vi "AOL Control-4ch.vi"() -> ()   [LabVIEW 2020]
uses:
  TypeDef/Frequency-4ch.ctl
  TypeDef/Amplitude-4ch.ctl
  TypeDef/FPGA_card_type.ctl
  TypeDef/FPGA_adapter_type.ctl
  Globals/FPGA Globals.vi
  <vilib>/DAQmx/create/channels.llb/DAQmx Create Channel (CO-Pulse Generation-Time).vi
panel:
  in  "Tab Control":T1(tab)
  out "Continuous Trigger  ON":bool
  in  "Tadj [us]":dbl
  in  "Tdwell [us]":dbl=0.4
  in  "AOD Fill":dbl=24.475
  in  "Ny":u16=39
  in  "Nx":u16=39
  in  "Use Cont. trigger":bool
  in  "Use RF from file":bool
  in  "RF Code File":path=path "D:/Microscope data/2019-04-16/Sameer/Packets"
  in  "Frequency (MHz)":T2={"Ch 1"=39, "Ch 2"=39, "Ch 3"=39, "Ch 4"=39} {"Ch 4" min=20 max=50 step=1; "Ch 3" min=20 max=50 step=1; "Ch 2" min=20 max=50 step=1; "Ch 1" min=20 max=50 step=1}
  in  "Amplitude":T3={"Ch 1"=255, "Ch 2"=255, "Ch 3"=255, "Ch 4"=255} {"Ch 4" max=255 step=1; "Ch 3" max=255 step=1; "Ch 2" max=255 step=1; "Ch 1" max=255 step=1}
  in  "Stop":bool
  in  "Load":bool
  in  "Run":bool
  in  "Clear":bool
  in  "Settings":bool
  out "Ethernet Port Opened":bool
  out "RF Loaded":bool
  out "Trigger Sent":bool
  out "Status":string
  in  "Use detected RIO resource":bool
  in  "RIO Resource Name":string
  out "Detected RIO Resource Name":string
  in  "Use FlexRIO Trigger":bool=TRUE
  in  "DAQmx Trigger Channel":tag="PXI1Slot4/ctr0"
  in  "Pulse Width (sec)":dbl=1e-05
  in  "Initial Delay(sec)":dbl=0.01 format="%.6f"
  in  "FPGA Card":T4
  in  "Adapter Module":T5
  out "task out":refnum<k21>
  out "PC Mac Address":string caption="PC MAC Address"
  out "Select Device 1":i32=1 caption="Device 1 Port" min=1 max=5 step=1
  out "Select Device 2":i32=1 caption="Device 2 Port" min=1 max=5 step=1
  out "Packet Array":string[](array[string])
  out "No of Packets":i32
  out "FPGA MAC 1":string caption="Device 1 MAC Address"
  out "FPGA MAC 2":string caption="Device 2 MAC Address"
  out "Trigger Error":errorcluster
  in  "error in":errorcluster
  # "User needs to send a single TTL rising edge for the controller to generate RF."
  # "Trigger"
  # "Ethernet"
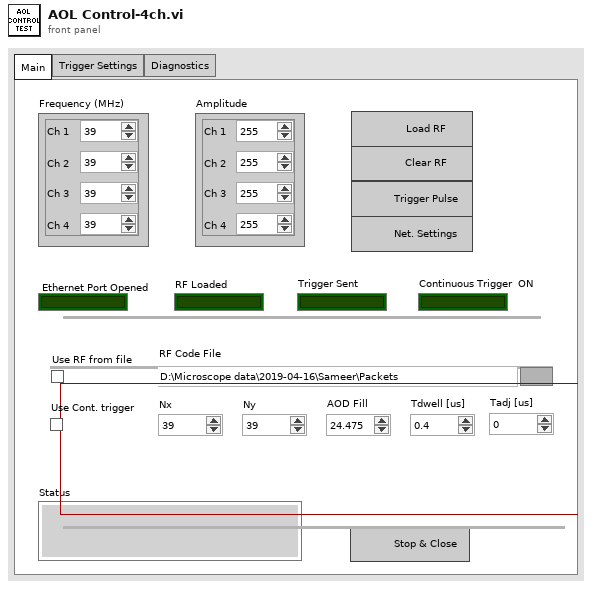
[diagram p1: front panel]
types:
  T1 = enum32{"Main", "Trigger Settings", "Diagnostics"}
  T2 = typedef "Frequency-4ch.ctl" = cluster{"Ch 1":u16, "Ch 2":u16, "Ch 3":u16, "Ch 4":u16}
  T3 = typedef "Amplitude-4ch.ctl" = cluster{"Ch 1":u16, "Ch 2":u16, "Ch 3":u16, "Ch 4":u16}
  T4 = typedef "FPGA_card_type.ctl" = enum16{"7976R", "7975R", "7966R"}
  T5 = typedef "FPGA_adapter_type.ctl" = enum16{"5772-DC", "5772-AC"}
  T6 = enum8{"Enabled", "Disabled", "Disabled and Grayed Out"}
  T7 = enum16{"Initialise FPGA ref", "Read FPGA ref", "Close FPGA Ref"}
  T8 = cluster{"Use FlexRIO Trigger":bool, "RIO Resource Name":string, "Use detected RIO resource":bool, "Ethernet Card WinPCap Port ":i16, "FPGA Card":string, "Adapter Module":string}
  T9 = typedef "FPGA_DAQ_settings.ctl" = cluster{"Use FlexRIO Trigger":bool, "RIO Resource Name":string, "Use detected RIO resource":bool, "Ethernet Card WinPCap Port ":i16, "Adapter Module":T5, "FPGA Card":T4}
  T10 = typedef "FPGA Settings.ctl" = cluster{"System Clock(MHz)":dbl, "FPGA MAC 1":string, "Port Number 1":i32, "Port Number 2":i32, "FPGA MAC 2":string, "PC MAC Address":string}
  T11 = cluster{"Pulse Period (us)":u32, "Pulse Width (us)":u32}
  T12 = typedef "FPGA_ref.ctl" = refnum<k20>
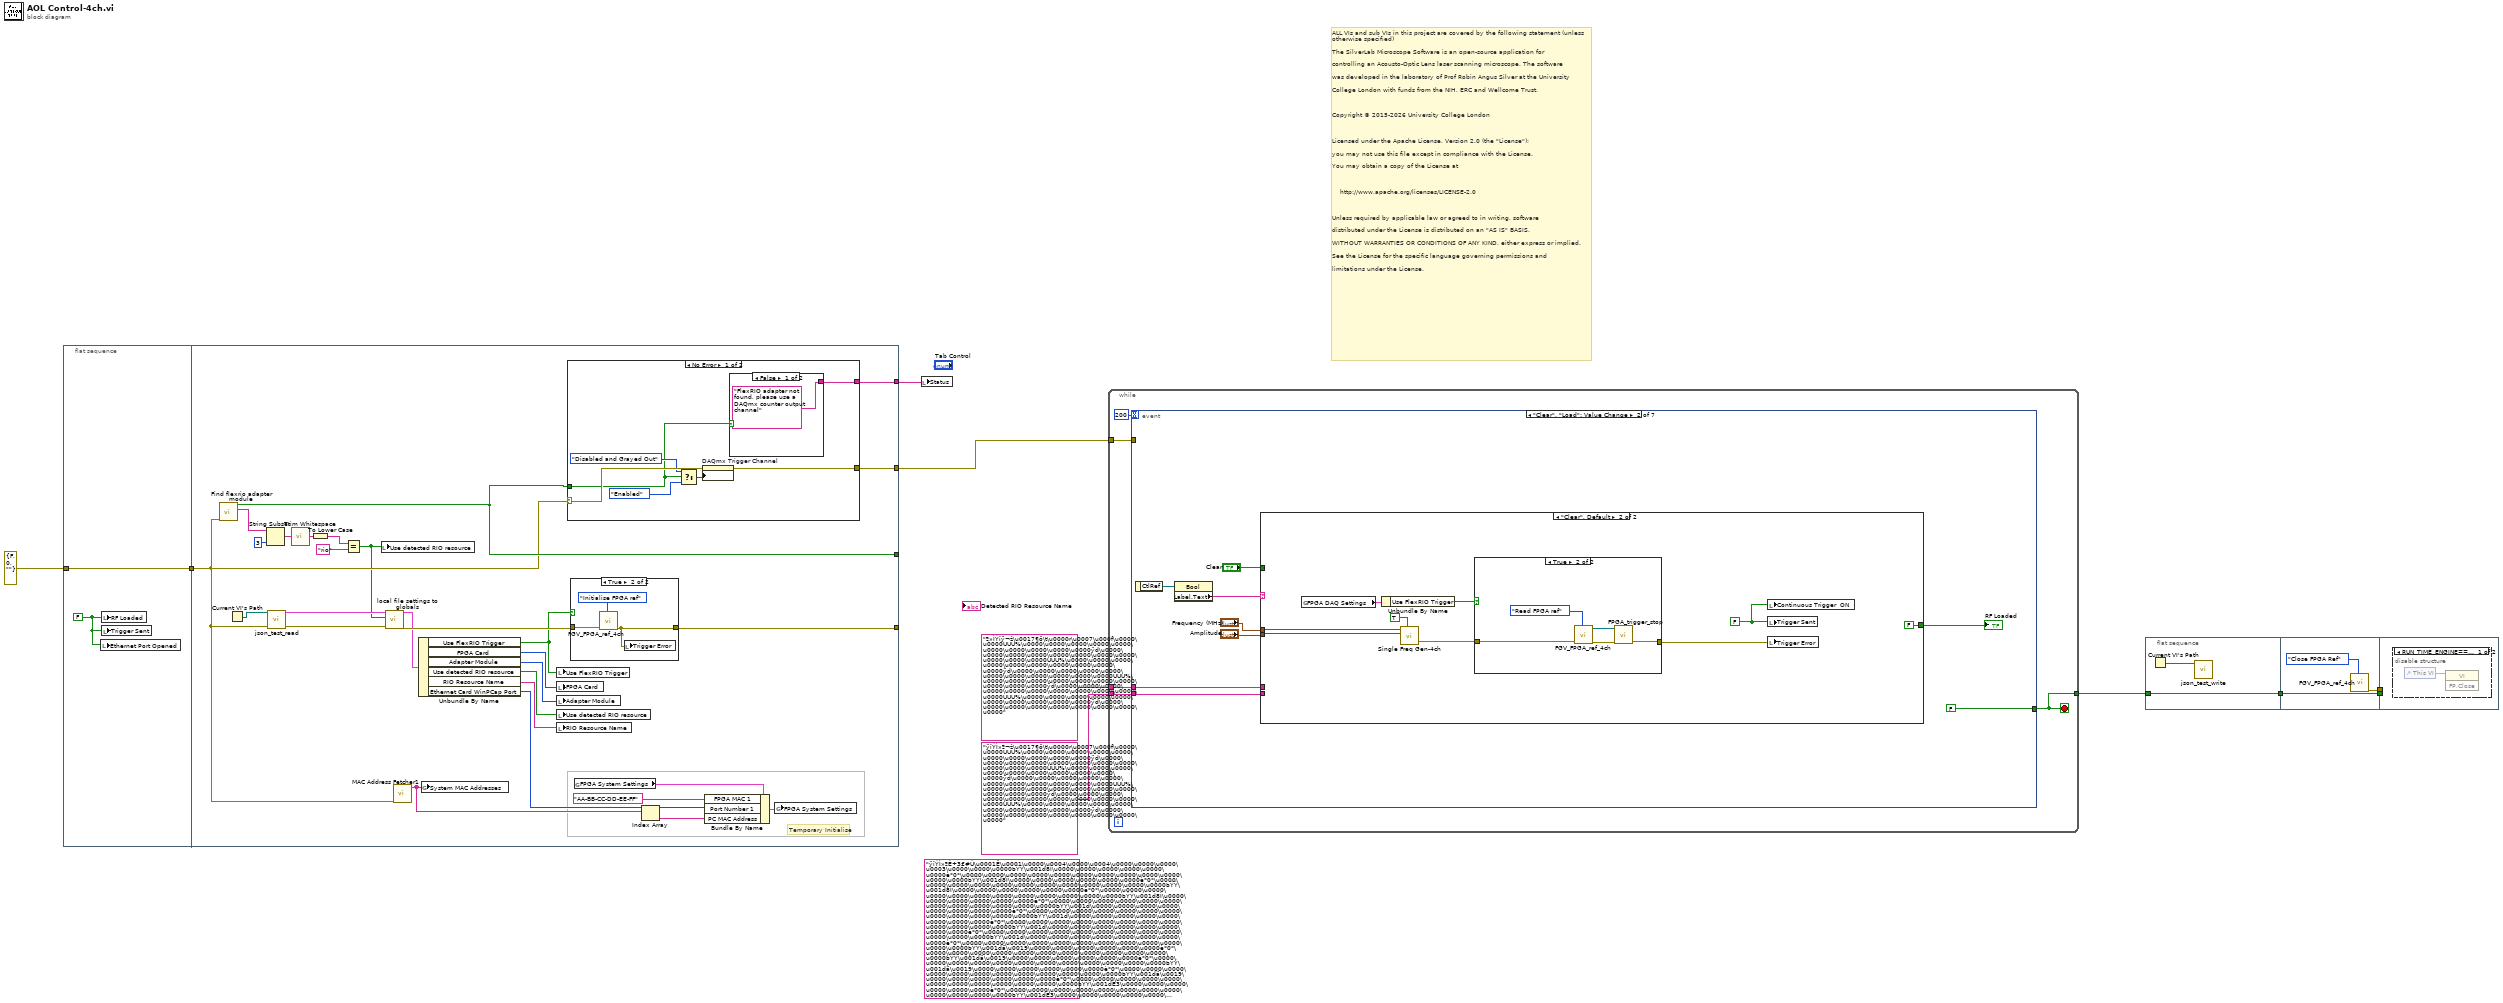
[diagram p0: block diagram]
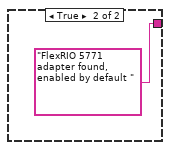
[diagram p2: hidden frame]
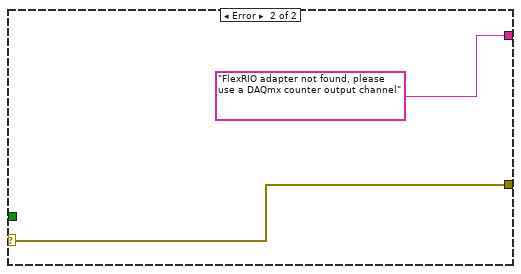
[diagram p3: hidden frame]
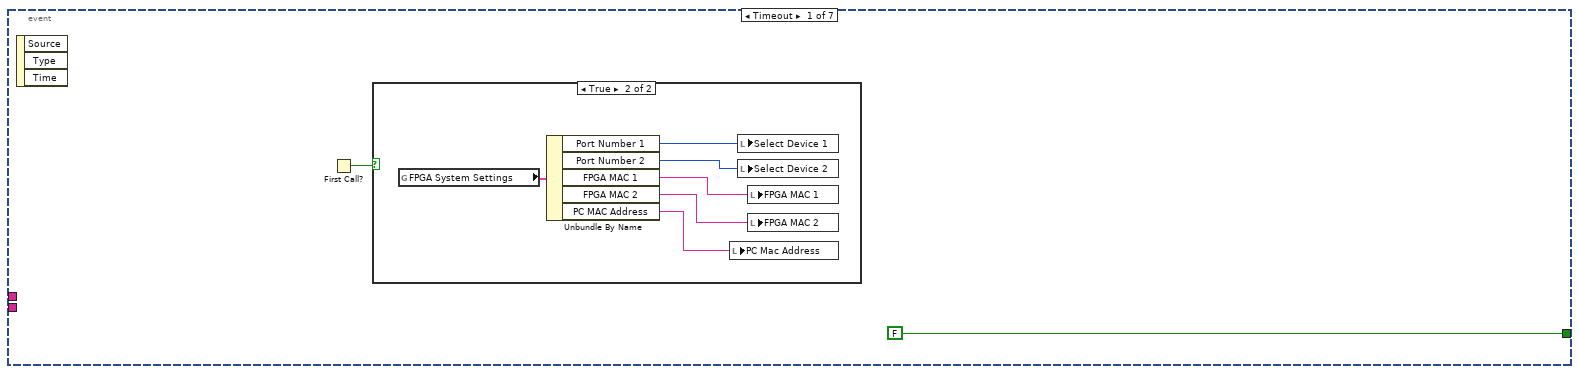
[diagram p6: hidden frame]
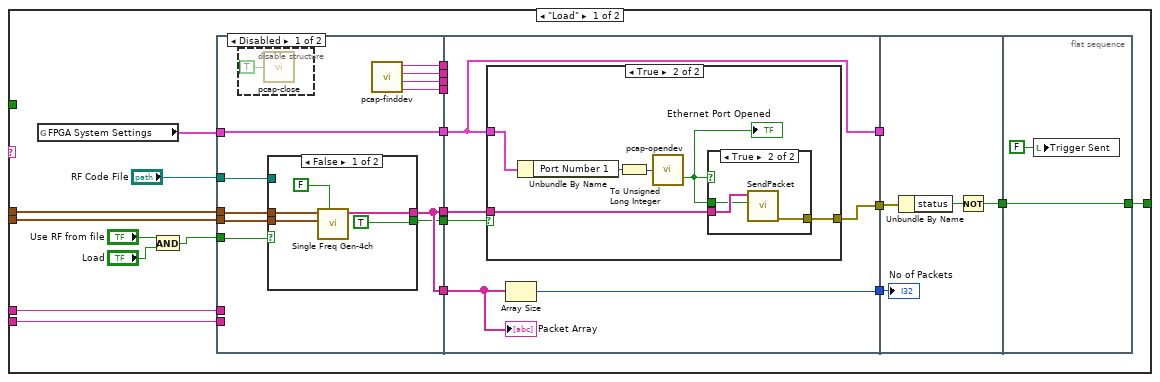
[diagram p8: hidden frame]
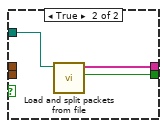
[diagram p9: hidden frame]
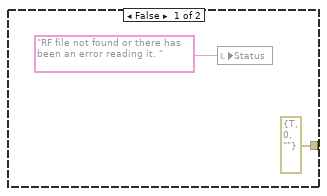
[diagram p11: hidden frame]
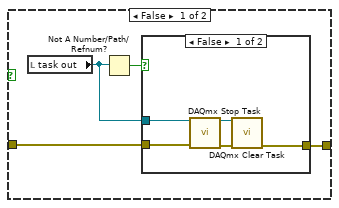
[diagram p13: hidden frame]
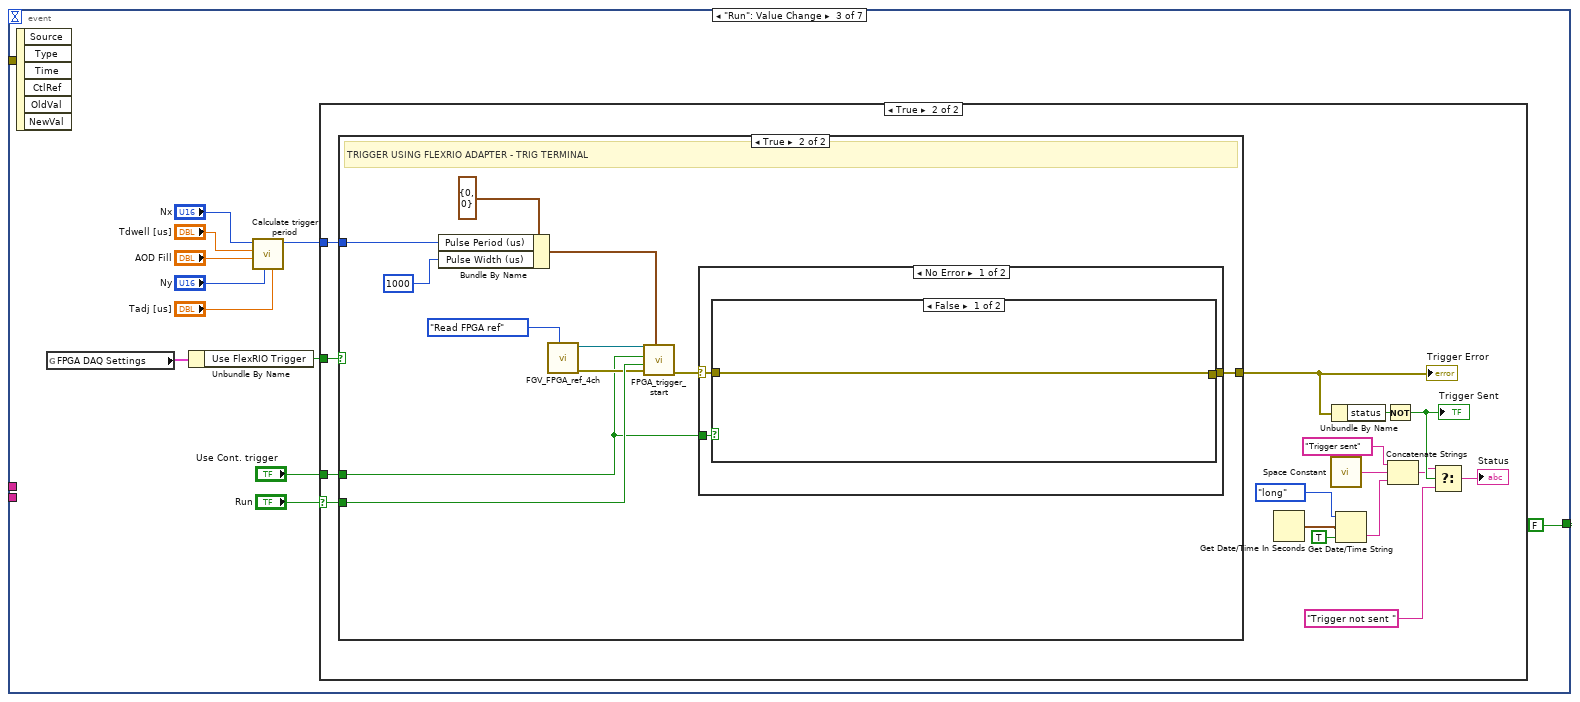
[diagram p15: hidden frame]
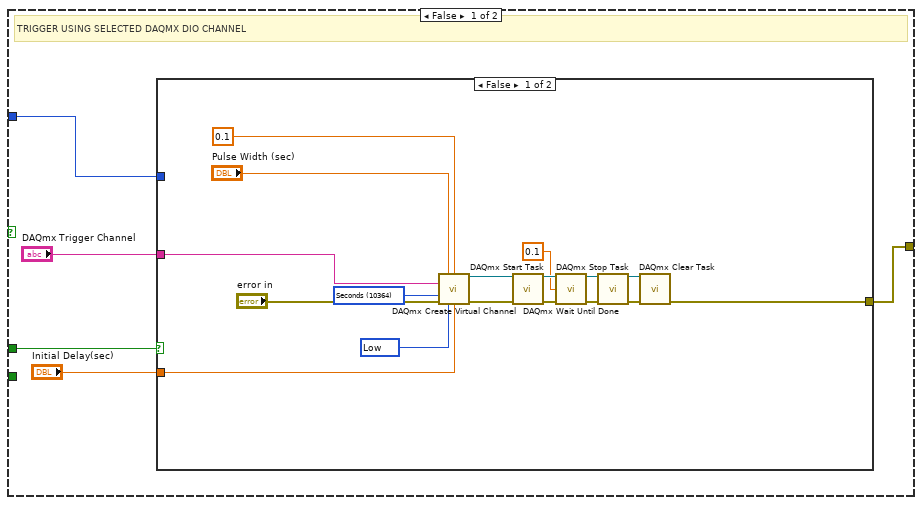
[diagram p17: hidden frame]
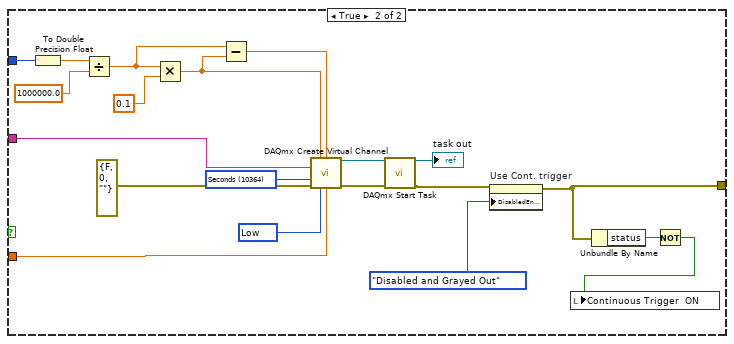
[diagram p18: hidden frame]
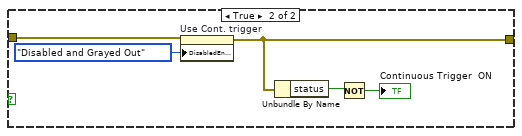
[diagram p19: hidden frame]
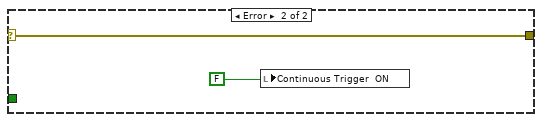
[diagram p20: hidden frame]
diagram:
  (unwired) "ÿîÝÌ»ªÈ÷3£#Ù\u0001Ê\u0001\u0000\u0004\u0000\u0004\u0000\u0000\u0000\u0003\u0000\u0000\u0000ÞÝÝ\u001d8Ì\u0000\u0000\u0000\u0000\u0000\u0000è*0*\u0000\u0000\u0000\u0000\u0000\u0000\u0000\u0000\u0000\u0000\u0000\u0000ÞÝÝ\u001d8Ì\u0000\u0000\u0000\u0000\u0000\u0000è*0*\u0000\u0000\u0000\u0000\u0000\u0000\u0000\u0000\u0000\u0000\u0000\u0000ÞÝÝ\u001d8Ì\u0000\u0000\u0000\u0000\u0000\u0000è*0*\u0000\u0000\u0000\u0000\u0000\u0000\u0000\u0000\u0000\u0000\u0000\u0000ÞÝÝ\u001d8Ì\u0000\u0000\u0000\u0000\u0000\u0000è*0*\u0000\u0000\u0000\u0000\u0000\u0000\u0000\u0000\u0000\u0000\u0000\u0000ÞÝÝ\u001d\u0000\u0000\u0000\u0000\u0000\u0000\u0000\u0000è*0*\u0000\u0000\u0000\u0000\u0000\u0000\u0000\u0000\u0000\u0000\u0000\u0000ÞÝÝ\u001d\u0000\u0000\u0000\u0000\u0000\u0000\u0000\u0000è*0*\u0000\u0000\u0000\u0000\u0000\u0000\u0000\u0000\u0000\u0000\u0000\u0000ÞÝÝ\u001d\u0000\u0000\u0000\u0000\u0000\u0000\u0000\u0000è*0*\u0000\u0000\u0000\u0000\u0000\u0000\u0000\u0000\u0000\u0000\u0000\u0000ÞÝÝ\u001d\u0000\u0000\u0000\u0000\u0000\u0000\u0000\u0000è*0*\u0000\u0000\u0000\u0000\u0000\u0000\u0000\u0000\u0000\u0000\u0000\u0000ÞÝÝ\u001dä\u0019\u0000\u0000\u0000\u0000\u0000\u0000è*0*\u0000\u0000\u0000\u0000\u0000\u0000\u0000\u0000\u0000\u0000\u0000\u0000ÞÝÝ\u001dä\u0019\u0000\u0000\u0000\u0000\u0000\u0000è*0*\u0000\u0000\u0000\u0000\u0000\u0000\u0000\u0000\u0000\u0000\u0000\u0000ÞÝÝ\u001dä\u0019\u0000\u0000\u0000\u0000\u0000\u0000è*0*\u0000\u0000\u0000\u0000\u0000\u0000\u0000\u0000\u0000\u0000\u0000\u0000ÞÝÝ\u001dä\u0019\u0000\u0000\u0000\u0000\u0000\u0000è*0*\u0000\u0000\u0000\u0000\u0000\u0000\u0000\u0000\u0000\u0000\u0000\u0000ÞÝÝ\u001dÈ3\u0000\u0000\u0000\u0000\u0000\u0000è*0*\u0000\u0000\u0000\u0000\u0000\u0000\u0000\u0000\u0000\u0000\u0000\u0000ÞÝÝ\u001dÈ3\u0000\u0000\u0000\u0000\u0000\u0000è*0*\u0000\u0000\u0000\u0000\u0000\u0000\u0000\u0000\u0000\u0000\u0000\u0000ÞÝÝ\u001dÈ3\u0000\u0000\u0000\u0000\u0000\u0000è*0*\u0000\u0000\u0000\u0000\u0000\u0000\u0000\u0000\u0000\u0000\u0000\u0000ÞÝÝ\u001dÈ3\u0000\u0000\u0000\u0000\u0000\u0000è*0*\u0000\u0000\u0000\u0000\u0000\u0000\u0000\u0000\u0000\u0000"
  # "ALL VIs and sub VIs in this project are covered by the following statement (unless \notherwise specified)\n\nThe SilverLab Microscope Software is an open-source application for\n\ncontrolling an Acousto-Optic Lens laser scanning microscope. The software\n\nwas developed in the laboratory of Prof Robin Angus Silver at the University\n\nCollege London with funds from the NIH, ERC and Wellcome Trust.\n\n \n\nCopyright © 2015-2026 University College London\n\n \n\nLicensed under the Apache License, Version 2.0 (the \"License\");\n\nyou may not use this file except in compliance with the License.\n\nYou may obtain a copy of the License at\n\n \n\n    http://www.apache.org/licenses/LICENSE-2.0\n\n \n\nUnless required by applicable law or agreed to in writing, software\n\ndistributed under the License is distributed on an \"AS IS\" BASIS,\n\nWITHOUT WARRANTIES OR CONDITIONS OF ANY KIND, either express or implied.\n\nSee the License for the specific language governing permissions and\n\nlimitations under the License."
  n1 = flat-sequence {
    tunnel: errorcluster {"status"=FALSE, "code"=0, "source"=""} ("error in (no error)") -> [w11]
    tunnel: [w11] -> w3
    tunnel: [w37] -> _
    tunnel: [w16] -> _
    tunnel: w3 -> [w15]
    tunnel: [w18] -> w2
    tunnel: [w17] -> w1
    frame #0 {
      w12 = FALSE ("RF Loaded")
      n2 = local write "Ethernet Port Opened"(w12) -> ()
      n3 = local write "RF Loaded"(w12) -> ()
      n4 = local write "Trigger Sent"(w12) -> ()
    }
    frame #1 {
      # "Temporary Initialise"
      n5 = call "Find flexrio adapter module.vi"("error in (no error)"=w15) -> ("Devices & Chassis:Provides Link Name"=w24:string, "NI 5772 adapter present ?"=w16:bool)  [unwired: 8 in, 1 out]
      n6 = Current VI's Path() -> (path=w13:path)
      n7 = String Subset(string=w24, length (rest)=3 ("length (rest)")) -> (substring=w23:string)  [unwired: 1 in]
      n8 = call "json_test_read.vi"("error in"=w15, "Parent VI Path"=w13) -> ("error out"=w39:errorcluster, "value"=w40:T8)  [unwired: 8 in]
      n9 = call <vilib>:"Trim Whitespace.vi"("string"=w23) -> ("trimmed string"=w22:string)  [unwired: 1 in]
      n10 = To Lower Case(string=w22) -> (all lower case string=w21:string)
      n11 = Equal?(x=w21, y="rio") -> (x = y?=w14:bool)
      n12 = local write "Use detected RIO resource"(w14) -> ()
      n13 = call "local file settings to globals.vi"("error in (no error)"=w39, "FPGA HW Detected"=w14, "DAQ FPGA Settings"=w40) -> ("error out"=w38:errorcluster, "DAQ FPGA Settings"=w36:T9)  [unwired: 7 in]
      n14 = call "MAC Address Fetcher1.vi"("error in (no error)"=w15) -> ("MAC Addresses"=w29:string[])  [unwired: 8 in, 2 out]
      n15 = Unbundle By Name(w36) -> ("Use FlexRIO Trigger"=w35:bool, "FPGA Card"=w34:T4, "Adapter Module"=w33:T5, "Use detected RIO resource"=w32:bool, "RIO Resource Name"=w25:string, "Ethernet Card WinPCap Port"=w26:i16)
      n16 = global write "FPGA Globals.vi" "System MAC Addresses"(w29) -> ()
      n17 = local write "Use FlexRIO Trigger"(w35) -> ()
      n18 = local write "FPGA Card"(w34) -> ()
      n19 = local write "Adapter Module"(w33) -> ()
      n20 = local write "Use detected RIO resource"(w32) -> ()
      n21 = local write "RIO Resource Name"(w25) -> ()
      n22 = case shown="No Error" w15 {
        selector: w15 -> [w47 w51]
        tunnel: w16 -> [w42 _]
        tunnel: [w43 w51] -> w18
        tunnel: [w41 "FlexRIO adapter not found, please use a DAQmx counter output channel"] -> w17
        frame No Error {
          n23 = Select(t=T6."Disabled and Grayed Out" ("Disabled"), s=w42, f=T6."Enabled") -> (s? t:f=w45:T6)
          n24 = property on="DAQmx Trigger Channel" class="DAQmxName"(error in=w47, "DisabledEnum"=w45) -> (error out=w43:errorcluster)  [unwired: 1 in, 1 out]
          n25 = case shown="False" w42 {
            tunnel: ["FlexRIO adapter not found, please use a DAQmx counter output channel" "FlexRIO 5771 adapter found, enabled by default "] -> w41
            frame False {
            }
            frame True {
            }
          }
        }
        frame Error {
        }
      }
      n26 = case shown="True" w35 {
        tunnel: w38 -> [w52 w55]
        tunnel: [w52 w53] -> w37
        frame False {
        }
        frame True {
          n27 = call "FGV_FPGA_ref_4ch.vi"("Action"=T7."Initialise FPGA ref", "error in (no error)"=w55) -> ("error out"=w53:errorcluster)  [unwired: 8 in, 1 out]
          n28 = local write "Trigger Error"(w53) -> ()
        }
      }
      n29 = global read "FPGA Globals.vi" "FPGA System Settings"() -> (w31:T10)
      n30 = Index Array(array=w29) -> (element=w28:string)  [unwired: 1 in]
      n31 = Bundle By Name(cluster=w31, "FPGA MAC 1"="AA-BB-CC-DD-EE-FF" ("FPGA MAC 3"), "Port Number 1"=w26, "PC MAC Address"=w28) -> (w30:T10)
      n32 = global write "FPGA Globals.vi" "FPGA System Settings"(w30) -> ()
    }
  }
  n33 = local write "Status"(w1) -> ()
  n34 = while {
    tunnel: "ª»ÌÝîÿ¬ž\u0017¶ö\t\u0000r\u0007\u000f\u0000\u0000UUU%\u0000\u0000\u0000\u0000\u0000\u0000\u0000\u0000\u0000\u0000ÿd\u0000\u0000\u0000\u0000\u0000\u0000\u0000\u0000\u0000\u0000\u0000UUU%\u0000\u0000\u0000\u0000\u0000\u0000\u0000\u0000\u0000\u0000ÿd\u0000\u0000\u0000\u0000\u0000\u0000\u0000\u0000\u0000\u0000\u0000UUU%\u0000\u0000\u0000\u0000\u0000\u0000\u0000\u0000\u0000\u0000ÿd\u0000\u0000\u0000\u0000\u0000\u0000\u0000\u0000\u0000\u0000\u0000UUU%\u0000\u0000\u0000\u0000\u0000\u0000\u0000\u0000\u0000\u0000ÿd\u0000\u0000\u0000\u0000\u0000\u0000\u0000\u0000\u0000" ("String") -> [w59]
    tunnel: "ÿîÝÌ»ª¬ž\u0017¶ö\t\u0000r\u0007\u000f\u0000\u0000UUU%\u0000\u0000\u0000\u0000\u0000\u0000\u0000\u0000\u0000\u0000ÿd\u0000\u0000\u0000\u0000\u0000\u0000\u0000\u0000\u0000\u0000\u0000UUU%\u0000\u0000\u0000\u0000\u0000\u0000\u0000\u0000\u0000\u0000ÿd\u0000\u0000\u0000\u0000\u0000\u0000\u0000\u0000\u0000\u0000\u0000UUU%\u0000\u0000\u0000\u0000\u0000\u0000\u0000\u0000\u0000\u0000ÿd\u0000\u0000\u0000\u0000\u0000\u0000\u0000\u0000\u0000\u0000\u0000UUU%\u0000\u0000\u0000\u0000\u0000\u0000\u0000\u0000\u0000\u0000ÿd\u0000\u0000\u0000\u0000\u0000\u0000\u0000\u0000\u0000" ("String") -> [w58]
    tunnel: [w57] -> w8
    tunnel: w2 -> [w56]
    stop <- w57 stop-if-true
    n35 = event shown="[1] \"Clear\", \"Load\": Value Change" {
      selector: _ -> [_ _ _ _ _ _ _]
      dyn-events: _ -> [_ _ _ _ _ _ _]
      timeout: 200 -> [_ _ _ _ _ _ _]
      tunnel: w59 -> [_ w76 _ _ _ _ _]
      tunnel: w58 -> [_ w75 _ _ _ _ _]
      tunnel: [FALSE FALSE FALSE _ _ FALSE w282] -> w57
      tunnel: w56 -> [_ _ _ _ _ _ _]
      event Timeout {
        n36 = event-data() -> ()  [unwired: 1 in, 3 out]
        n37 = First Call?() -> (First Call?: T/F=w61:bool)
        n38 = case shown="True" w61 {
          frame False {
          }
          frame True {
            n39 = global read "FPGA Globals.vi" "FPGA System Settings"() -> (w68:T10)
            n40 = Unbundle By Name(w68) -> ("Port Number 1"=w67:i32, "Port Number 2"=w66:i32, "FPGA MAC 1"=w65:string, "FPGA MAC 2"=w64:string, "PC MAC Address"=w63:string)
            n41 = local write "PC Mac Address"(w63) -> ()
            n42 = local write "Select Device 1"(w67) -> ()
            n43 = local write "Select Device 2"(w66) -> ()
            n44 = local write "FPGA MAC 1"(w65) -> ()
            n45 = local write "FPGA MAC 2"(w64) -> ()
          }
        }
      }
      event "Clear", "Load": Value Change {
        n46 = event-data() -> ("CtlRef"=w72:refnum<vi>)  [unwired: 1 in]
        n47 = property class="Bool"(reference=w72) -> ("Label.Text"=w71:string)  [unwired: 1 in, 2 out]
        n48 = case shown="\"Clear\", Default" w71 {
          tunnel: "Clear" -> [_ _]
          tunnel: w76 -> [w90 _]
          tunnel: w75 -> [w89 _]
          tunnel: [w87 FALSE] -> w73
          tunnel: "Frequency (MHz)" -> [w79 w150]
          tunnel: "Amplitude" -> [w78 w149]
          frame "Load" {
            n49 = global read "FPGA Globals.vi" "FPGA System Settings"() -> (w95:T10)
            n50 = And(x="Use RF from file", y="Load") -> (x .and. y?=w80:bool)
            n51 = flat-sequence {
              tunnel: w78 -> [w110]
              tunnel: w79 -> [w109]
              tunnel: [w108] -> w99
              tunnel: w95 -> [w108]
              tunnel: [w107] -> w94
              tunnel: [w106] -> w93
              tunnel: [w105] -> w92
              tunnel: [w104] -> w91
              tunnel: w90 -> [_]
              tunnel: w89 -> [_]
              tunnel: [w103] -> w88
              tunnel: [w103] -> w85
              tunnel: w80 -> [w102]
              tunnel: "RF Code File" -> [w101]
              tunnel: [w100] -> w83
              tunnel: [w125] -> w98
              tunnel: [w124] -> w97
              tunnel: w99 -> [w123]
              tunnel: [w123] -> w96
              tunnel: w94 -> [_]
              tunnel: w93 -> [_]
              tunnel: w92 -> [_]
              tunnel: w91 -> [_]
              tunnel: w88 -> [w122]
              tunnel: w85 -> [w121]
              tunnel: w83 -> [w120]
              tunnel: w98 -> [w139]
              tunnel: w97 -> [w140]
              tunnel: w96 -> [_]
              tunnel: [w137] -> w86
              tunnel: [w142] -> w87
              tunnel: w86 -> [w142]
              frame #0 {
                n52 = disable-structure shown="Disabled" {
                  frame Disabled {
                    n53 = call "pcap-close.vi"("Opened"=TRUE) -> ()
                  }
                  frame Enabled {
                  }
                }
                n54 = case shown="False" w102 {
                  tunnel: w110 -> [w115 _]
                  tunnel: w109 -> [w114 _]
                  tunnel: [w113 w116] -> w103
                  tunnel: w101 -> [_ w118]
                  tunnel: [TRUE ("OK?") w117] -> w100
                  frame False {
                    n55 = call "Single Freq Gen-4ch.vi"("Stop Single Frquency"=FALSE, "Amplitude"=w115, "Frequency (MHz)"=w114) -> ("Hex String (Array)"=w113:string[])  [unwired: 7 in, 1 out]
                  }
                  frame True {
                    n56 = call "Load and split packets from file.vi"("Path"=w118) -> ("OK?"=w117:bool, "Hex String"=w116:string[])  [unwired: 7 in, 2 out]
                  }
                }
                n57 = call "pcap-finddev.vi"() -> ("String 4"=w104:string, "String 3"=w105:string, "String 2"=w106:string, "String"=w107:string)  [unwired: 1 in, 1 out]
              }
              frame #1 {
                n58 = case shown="True" w120 {
                  tunnel: [errorcluster {"status"=TRUE, "code"=0, "source"=""} ("error out") w133] -> w125
                  tunnel: w123 -> [_ w130]
                  tunnel: w122 -> [_ w128]
                  frame False {
                    n59 = local write "Status"("RF file not found or there has been an error reading it. " ("Status")) -> ()
                  }
                  frame True {
                    n60 = Unbundle By Name(w130) -> ("Port Number 1"=w132:i32)
                    n61 = To Unsigned Long Integer(number=w132) -> (unsigned 32bit integer=w131:u32)
                    n62 = call "pcap-opendev.vi"("Select Device"=w131) -> ("Opened"=w129:bool)  [unwired: 2 out]
                    "Ethernet Port Opened" <- w129
                    n63 = case shown="True" w129 {
                      tunnel: [_ w136] -> w133
                      tunnel: w128 -> [_ w135]
                      tunnel: w129 -> [_ w134]
                      frame False {
                      }
                      frame True {
                        n64 = call "SendPacket.vi"("Ethernet Port Opened ?"=w134, "Packet Array"=w135) -> ("error out"=w136:errorcluster)  [unwired: 8 in, 1 out]
                      }
                    }
                  }
                }
                n65 = Array Size(array=w121) -> (size(s)=w124:i32)
                "Packet Array" <- w121
              }
              frame #2 {
                n66 = Unbundle By Name(w139) -> ("status"=w138:bool)
                n67 = Not(x=w138) -> (.not. x?=w137:bool)
                "No of Packets" <- w140
              }
              frame #3 {
                n68 = local write "Trigger Sent"(FALSE ("Trigger Sent")) -> ()
              }
            }
          }
          frame "Clear", Default {
            w143 = FALSE ("Trigger Sent")
            n69 = global read "FPGA Globals.vi" "FPGA DAQ Settings"() -> (w146:T9)
            n70 = Unbundle By Name(w146) -> ("Use FlexRIO Trigger"=w145:bool)
            n71 = call "Single Freq Gen-4ch.vi"("Stop Single Frquency"=TRUE, "Amplitude"=w149, "Frequency (MHz)"=w150) -> ("error out"=w148:errorcluster)  [unwired: 7 in, 1 out]
            n72 = case shown="True" w145 {
              tunnel: w148 -> [w154 w165]
              tunnel: [w152 w162] -> w144
              frame False {
                n73 = local read "task out"() -> (w153:refnum<k21>)
                n74 = Not A Number/Path/Refnum?(number/path/refnum=w153) -> (NaN/Path/Refnum?=w155:bool)
                n75 = case shown="False" w155 {
                  tunnel: w154 -> [w158 w161]
                  tunnel: w153 -> [w157 _]
                  tunnel: [w156 w161] -> w152
                  frame False {
                    n76 = call <vilib>:"DAQmx Stop Task.vi"("task/channels in"=w157, "error in"=w158) -> ("task out"=w160:refnum<k21>, "error out"=w159:errorcluster)  [unwired: 12 in]
                    n77 = call <vilib>:"DAQmx Clear Task.vi"("task in"=w160, "error in"=w159) -> ("error out"=w156:errorcluster)  [unwired: 13 in]
                  }
                  frame True {
                  }
                }
              }
              frame True {
                n78 = call "FGV_FPGA_ref_4ch.vi"("Action"=T7."Read FPGA ref", "error in (no error)"=w165) -> ("error out"=w164:errorcluster, "FPGA VI Reference Out"=w163:T12)  [unwired: 8 in]
                n79 = call "FPGA_trigger_stop.vi"("error in (no error)"=w164, "FPGA VI Reference IN"=w163) -> ("error out"=w162:errorcluster)  [unwired: 8 in, 1 out]
              }
            }
            n80 = local write "Continuous Trigger  ON"(w143) -> ()
            n81 = local write "Trigger Sent"(w143) -> ()
            n82 = local write "Trigger Error"(w144) -> ()
          }
        }
        "RF Loaded" <- w73
      }
      event "Run": Value Change {
        n83 = event-data() -> ()  [unwired: 1 in, 6 out]
        n84 = global read "FPGA Globals.vi" "FPGA DAQ Settings"() -> (w174:T9)
        n85 = Unbundle By Name(w174) -> ("Use FlexRIO Trigger"=w173:bool)
        n86 = call "Calculate trigger period.vi"("Tadj [us]"="Tadj [us]", "Ny"="Ny", "AOD Fill"="AOD Fill", "Tdwell [us]"="Tdwell [us]", "Nx"="Nx") -> ("period"=w168:u32)  [unwired: 6 in]
        n87 = case shown="True" "Run" {
          selector: "Run" -> [_ w188]
          tunnel: "Use Cont. trigger" -> [_ w187]
          tunnel: w173 -> [_ w186]
          tunnel: w168 -> [_ w185]
          frame False {
          }
          frame True {
            n88 = case shown="True" w186 {
              tunnel: [w198 w237] -> w193
              tunnel: w188 -> [_ w243]
              tunnel: w187 -> [w197 w236]
              tunnel: w185 -> [w195 w239]
              frame False {
                # "TRIGGER USING SELECTED DAQMX DIO CHANNEL"
                n89 = case shown="False" w197 {
                  tunnel: [w203 w218] -> w198
                  tunnel: "DAQmx Trigger Channel" -> [w202 w233]
                  tunnel: w195 -> [_ w231]
                  tunnel: "Initial Delay(sec)" -> [w200 w227]
                  frame False {
                    w199 = 10364 items=["Seconds"=10364] ("units")
                    w201 = 10214 items=["High"=10192, "Low"=10214] ("idle state")
                    n90 = call-poly <vilib>:"DAQmx Create Virtual Channel.vi"("high time"="Pulse Width (sec)", "low time"=0.1 ("Pulse Low Time(sec)"), "counter"=w202, "units"=w199, "error in"="error in", "idle state"=w201, "initial delay"=w200) -> ("task out"=w212:refnum<k21>, "error out"=w211:errorcluster)  [unwired: 7 in]
                    n91 = call <vilib>:"DAQmx Start Task.vi"("task/channels in"=w212, "error in"=w211) -> ("task out"=w210:refnum<k21>, "error out"=w206:errorcluster)  [unwired: 12 in]
                    n92 = call <vilib>:"DAQmx Wait Until Done.vi"("task/channels in"=w210, "timeout (sec)"=0.1, "error in"=w206) -> ("task out"=w205:refnum<k21>, "error out"=w204:errorcluster)  [unwired: 11 in]
                    n93 = call <vilib>:"DAQmx Stop Task.vi"("task/channels in"=w205, "error in"=w204) -> ("task out"=w209:refnum<k21>, "error out"=w208:errorcluster)  [unwired: 12 in]
                    n94 = call <vilib>:"DAQmx Clear Task.vi"("task in"=w209, "error in"=w208) -> ("error out"=w203:errorcluster)  [unwired: 13 in]
                  }
                  frame True {
                    w226 = 10364 items=["Seconds"=10364] ("units")
                    w228 = 10214 items=["High"=10192, "Low"=10214] ("idle state")
                    n95 = To Double Precision Float(number=w231) -> (double precision float=w230:dbl)
                    n96 = Divide(x=w230, y=1000000.0) -> (x/y=w224:dbl)
                    n97 = Multiply(x=w224, y=0.1) -> (x*y=w223:dbl)
                    n98 = Subtract(x=w224, y=w223) -> (x-y=w222:dbl)
                    n99 = call-poly <vilib>:"DAQmx Create Virtual Channel.vi"("high time"=w223, "low time"=w222, "counter"=w233, "units"=w226, "error in"=errorcluster {"status"=FALSE, "code"=0, "source"=""}, "idle state"=w228, "initial delay"=w227) -> ("task out"=w235:refnum<k21>, "error out"=w234:errorcluster)  [unwired: 7 in]
                    n100 = call <vilib>:"DAQmx Start Task.vi"("task/channels in"=w235, "error in"=w234) -> ("task out"=→"task out":refnum<k21>, "error out"=w219:errorcluster)  [unwired: 12 in]
                    n101 = property on="Use Cont. trigger" class="Bool (strict)"(error in=w219, "DisabledEnum"=T6."Disabled and Grayed Out" ("Disabled")) -> (error out=w218:errorcluster)  [unwired: 1 in, 1 out]
                    n102 = Unbundle By Name(w218) -> ("status"=w217:bool)
                    n103 = Not(x=w217) -> (.not. x?=w216:bool)
                    n104 = local write "Continuous Trigger  ON"(w216) -> ()
                  }
                }
              }
              frame True {
                # "TRIGGER USING FLEXRIO ADAPTER - TRIG TERMINAL"
                n105 = Bundle By Name(cluster=T11 {"Pulse Period (us)"=0, "Pulse Width (us)"=0} ("Pulse params"), "Pulse Period (us)"=w239, "Pulse Width (us)"=u32 1000) -> (w244:T11)
                n106 = call "FGV_FPGA_ref_4ch.vi"("Action"=T7."Read FPGA ref") -> ("error out"=w241:errorcluster, "FPGA VI Reference Out"=w240:T12)  [unwired: 9 in]
                n107 = call "FPGA_trigger_start.vi"("Pulse params"=w244, "error in"=w241, "TL Input"=w243, "Use Cont. trigger"=w236, "FPGA VI Reference IN"=w240) -> ("error out"=w238:errorcluster)  [unwired: 6 in]
                n108 = case shown="No Error" w238 {
                  selector: w238 -> [w249 w257]
                  tunnel: [w248 w257] -> w237
                  tunnel: w236 -> [w247 _]
                  frame No Error {
                    n109 = case shown="False" w247 {
                      tunnel: w249 -> [w250 w255]
                      tunnel: [w250 w253] -> w248
                      frame False {
                      }
                      frame True {
                        n110 = property on="Use Cont. trigger" class="Bool (strict)"(error in=w255, "DisabledEnum"=T6."Disabled and Grayed Out" ("Disabled")) -> (error out=w253:errorcluster)  [unwired: 1 in, 1 out]
                        n111 = Unbundle By Name(w253) -> ("status"=w252:bool)
                        n112 = Not(x=w252) -> (.not. x?=→"Continuous Trigger  ON":bool)
                      }
                    }
                  }
                  frame Error {
                    n113 = local write "Continuous Trigger  ON"(FALSE) -> ()
                  }
                }
              }
            }
            "Trigger Error" <- w193
            n114 = Get Date/Time In Seconds() -> (seconds since 1Jan1904=w182:timestamp)
            n115 = call <vilib>:"Space Constant.vi"() -> ("String"=w180:string)
            n116 = Unbundle By Name(w193) -> ("status"=w192:bool)
            n117 = Get Date/Time String(date format (0)=enum16{"short", "long", "abbreviated"}."long", seconds (now)=w182, want seconds? (F)=TRUE) -> (time string=w179:string)  [unwired: 1 out]
            n118 = Not(x=w192) -> (.not. x?=w191:bool)
            "Trigger Sent" <- w191
            n119 = Concatenate Strings("Trigger sent", w180, w179) -> (w183:string)
            n120 = Select(t=w183, s=w191, f="Trigger not sent ") -> (s? t:f=→"Status":string)
          }
        }
      }
      event "Use FlexRIO Trigger": Value Change {
        n121 = event-data() -> ("NewVal"=w258:bool)  [unwired: 1 in, 5 out]
        n122 = global read "FPGA Globals.vi" "FPGA DAQ Settings"() -> (w260:T9)
        n123 = Select(t=T6."Disabled and Grayed Out" ("Disabled"), s=w258, f=T6."Enabled" ("Disabled")) -> (s? t:f=w261:T6)
        n124 = Bundle By Name(cluster=w260, "Use FlexRIO Trigger"=w258) -> (w259:T9)
        n125 = property on="DAQmx Trigger Channel" class="DAQmxName"("DisabledEnum"=w261) -> ()  [unwired: 2 in, 2 out]
        n126 = global write "FPGA Globals.vi" "FPGA DAQ Settings"(w259) -> ()
        n127 = case shown="True" w258 {
          frame False {
          }
          frame True {
            n128 = call "FGV_FPGA_ref_4ch.vi"("Action"=T7."Initialise FPGA ref") -> ("error out"=w264:errorcluster)  [unwired: 9 in, 1 out]
            n129 = local write "Trigger Error"(w264) -> ()
          }
        }
      }
      event "Use detected RIO resource", "RIO Resource Name": Value Change {
        n130 = event-data() -> ()  [unwired: 1 in, 6 out]
        n131 = flat-sequence {
          frame #0 {
            n132 = global read "FPGA Globals.vi" "FPGA DAQ Settings"() -> (w271:T9)
            n133 = Bundle By Name(cluster=w271, "FPGA Card"="FPGA Card", "Adapter Module"="Adapter Module", "Use detected RIO resource"="Use detected RIO resource", "RIO Resource Name"="RIO Resource Name") -> (w268:T9)
            n134 = global write "FPGA Globals.vi" "FPGA DAQ Settings"(w268) -> ()
          }
          frame #1 {
            n135 = call "FGV_FPGA_ref_4ch.vi"("Action"=T7."Initialise FPGA ref") -> ("error out"=w272:errorcluster)  [unwired: 9 in, 1 out]
            n136 = local write "Trigger Error"(w272) -> ()
          }
        }
      }
      event "Settings": Value Change {
        n137 = event-data() -> ()  [unwired: 1 in, 6 out]
        n138 = case shown="True" "Settings" {
          frame False {
          }
          frame True {
            n139 = flat-sequence {
              frame #0 {
                n140 = call "FPGA Selection.vi"() -> ()  [unwired: 12 in]
              }
              frame #1 {
                n141 = global read "FPGA Globals.vi" "FPGA System Settings"() -> (w279:T10)
                n142 = Unbundle By Name(w279) -> ("Port Number 1"=→"Select Device 1":i32, "Port Number 2"=→"Select Device 2":i32, "FPGA MAC 1"=→"FPGA MAC 1":string, "FPGA MAC 2"=→"FPGA MAC 2":string, "PC MAC Address"=→"PC Mac Address":string)
              }
            }
          }
        }
      }
      event "Stop": Value Change {
        n143 = event-data() -> ()  [unwired: 1 in, 6 out]
        n144 = local read "Ethernet Port Opened"() -> (w283:bool)
        n145 = flat-sequence {
          tunnel: w283 -> [w285]
          tunnel: [TRUE] -> w282
          frame #0 {
            n146 = call "pcap-close.vi"("Opened"=w285) -> ()
          }
        }
      }
    }
  }
  n147 = flat-sequence {
    tunnel: w8 -> [w287]
    tunnel: [w287] -> w4
    tunnel: [w290] -> w6
    tunnel: [w288] -> w5
    tunnel: w4 -> [w290]
    tunnel: w6 -> [_]
    tunnel: w5 -> [_]
    frame #0 {
      n148 = Current VI's Path() -> (path=w286:path)
      n149 = call "json_test_write.vi"("Application Directory"=w286) -> ()  [unwired: 11 in]
    }
    frame #1 {
      n150 = call "FGV_FPGA_ref_4ch.vi"("Action"=T7."Close FPGA Ref") -> ("error out"=w288:errorcluster)  [unwired: 9 in, 1 out]
    }
    frame #2 {
      n151 = disable-structure shown="RUN_TIME_ENGINE==True" {
        frame condition #0 {
          n152 = control-ref of="This VI"() -> (w291:refnum<vi>)
          n153 = invoke class="VI" method="FP.Close"(reference=w291) -> ()  [unwired: 2 in, 3 out]
        }
        frame condition #1 (active) {
        }
      }
    }
  }
